vi "Read Sub Panel coin.vi"(8 "error in (no error)":errorcluster, 11 "MXN actor in":refnum<class "MXN actor.lvclass">) -> (0 "error out":errorcluster, 2 "Sub Panel coin":refnum<vi>, 3 "MXN actor out":refnum<class "MXN actor.lvclass">)   [LabVIEW 2020, in "MXN actor.lvlib" / "MXN actor.lvclass"]
uses:
  MXN actor.lvclass
  MXN actor.lvclass/MXN actor.ctl
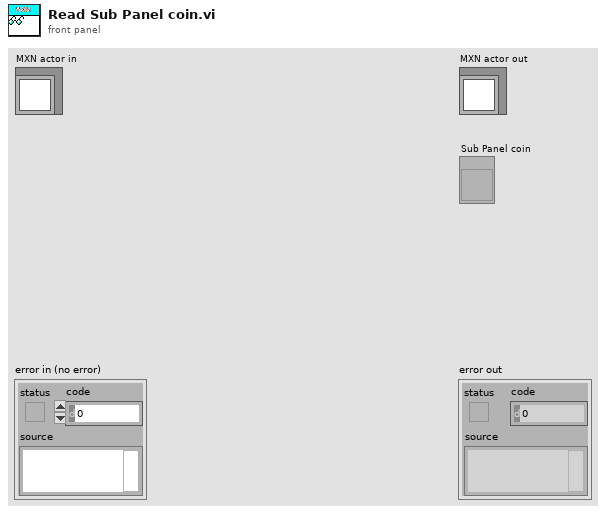
[diagram p1: front panel]
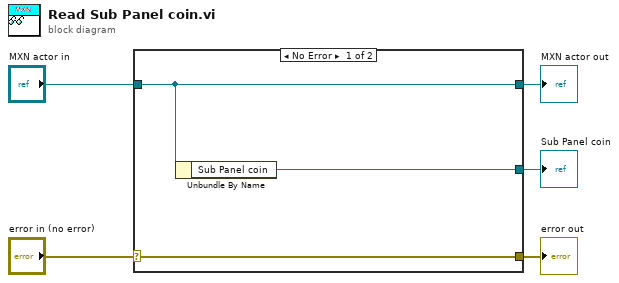
[diagram p0: block diagram]
diagram:
  n1 = case shown="No Error" "error in (no error)" {
    selector: "error in (no error)" -> [w8 w9]
    tunnel: [w8 w9] -> w4
    tunnel: [w7 w10] -> w2
    tunnel: "MXN actor in" -> [w7 w10]
    tunnel: [w6 _] -> w1
    frame No Error {
      n2 = Unbundle By Name(w7) -> ("Sub Panel coin"=w6:refnum<vi>)
    }
    frame Error {
    }
  }
  "error out" <- w4
  "MXN actor out" <- w2
  "Sub Panel coin" <- w1
